vi "Kinesis - KNA - Set Phase Component.vi"() -> ()   [LabVIEW 2012]
doc: "This VI shows how to set and get the phase comp."
uses:
  C:/Users/bhallewell/Desktop/Kinesis_with_LabVIEW_Examples_LV12_v1/Thorlabs.MotionControl.Controls.dll
  Thorlabs.MotionControl.Controls.dll
  C:/Users/bhallewell/Desktop/Kinesis_with_LabVIEW_Examples_LV12_v1/Thorlabs.MotionControl.KCube.NanoTrakCLI.dll
  Thorlabs.MotionControl.KCube.NanoTrakCLI.dll
  C:/Users/bhallewell/Desktop/Kinesis_with_LabVIEW_Examples_LV12_v1/Thorlabs.MotionControl.GenericNanoTrakCLI.dll
  Thorlabs.MotionControl.GenericNanoTrakCLI.dll
panel:
  in  "?":bool
  in  "KCubeNanoTrakControl":refnum<k24>(container)
  out "New Params":cluster{"HComponent":dbl, "VComponent":dbl}
  out "Initial Params":cluster{"HComponent":dbl, "VComponent":dbl}
  in  "Set Phase Compensation Parameters":bool
  in  "Set Params":cluster{"HComponent ":dbl, "VComponent":dbl}
  in  "SerialNumber":string
  # "Notes:"
  # "- Ensure that the appropriate .DLLs are copied into your Project Folder. Check that the correct bit type are used depending on your version of LabVIEW\ni.e. 32-bit or 64-bit.\n\n\n\n\n\n\n\n\n\n\n\n\n\n\n- Open the example VI through the LabVIEW Project Explorer to correctly load the User Interface from Thorlabs.MotionControl.Controls.dll."
  # "Thorlabs Hardware: KNA - K-Cube Nanotrak Controller\nhttps://www.thorlabs.com/newgrouppage9.cfm?objectgroup_id=2877"
  # "This VI will enable you to run the Kinesis Device panel for KNA-nnn devices. \nYou will also be set the H- & V-Components of the Phase Compensation or Angle of the Circle Path.\n\n1. Connect your KNA-nnn device to your PC via USB & power your device.\n2. Enter the serial number of the controller into the SerialNumber box below.\n3. Run the VI"
  # "Example Image of .NET Controller - VI opened via Project Explorer/ not opened via Project Explorer"
  # "VI Not Opened via Project Explorer"
  # "VI Opened via Project Explorer"
  # "- To explore the range of methods available, please visit the .NET API, included with your Kinesis software.\n\n- For tips on building your own VIs with Thorlabs Motion Control Hardware, please see our LabVIEW Guide here.\nhttps://www.thorlabs.com/newgrouppage9.cfm?objectgroup_id=10285"
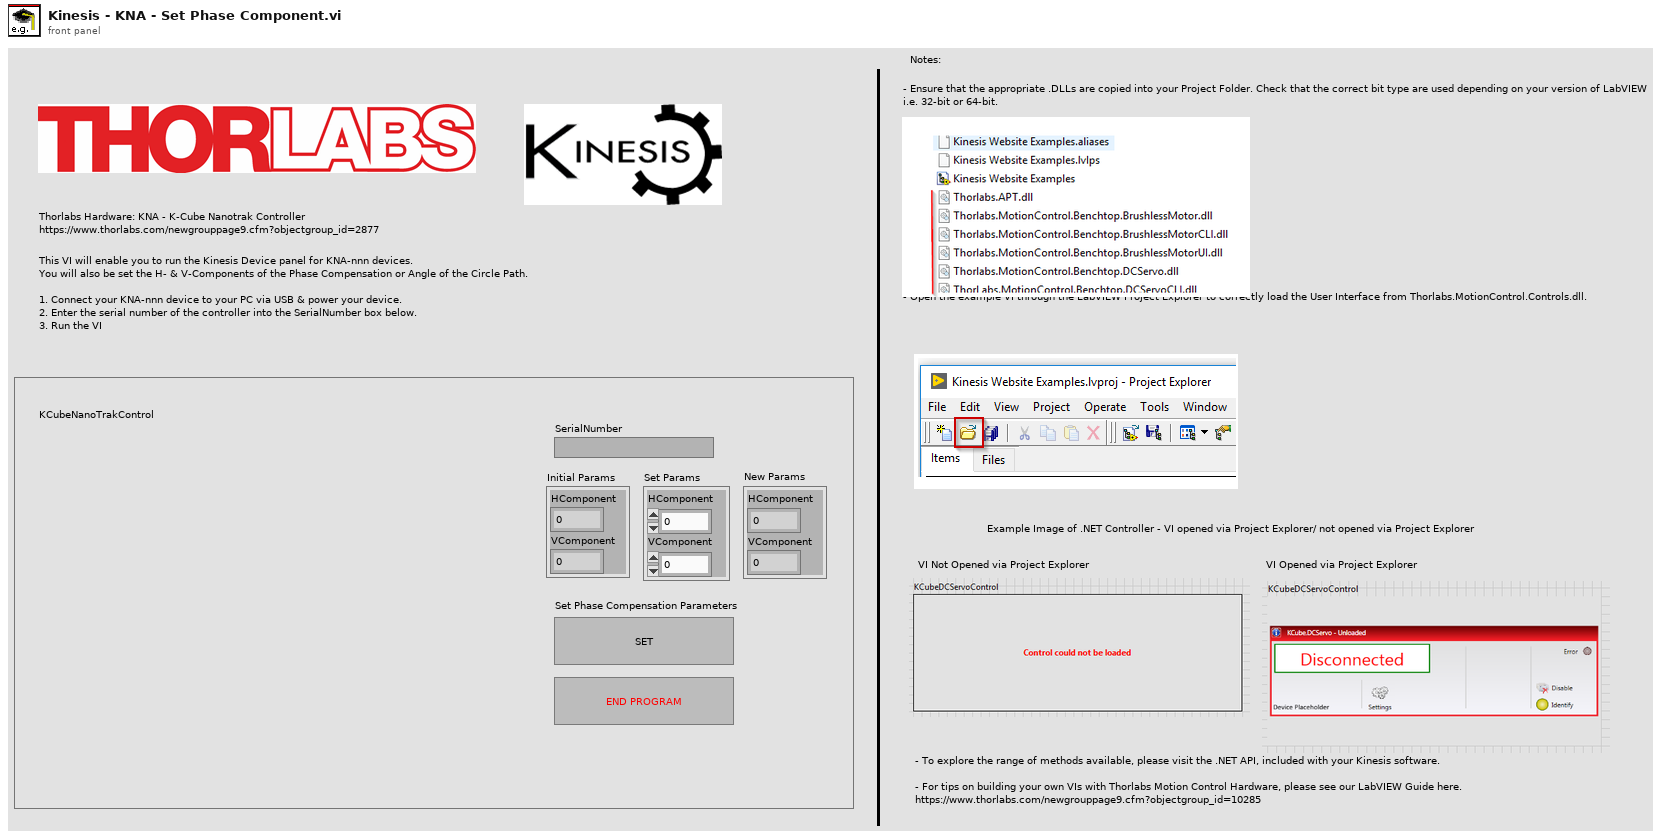
[diagram p1: front panel]
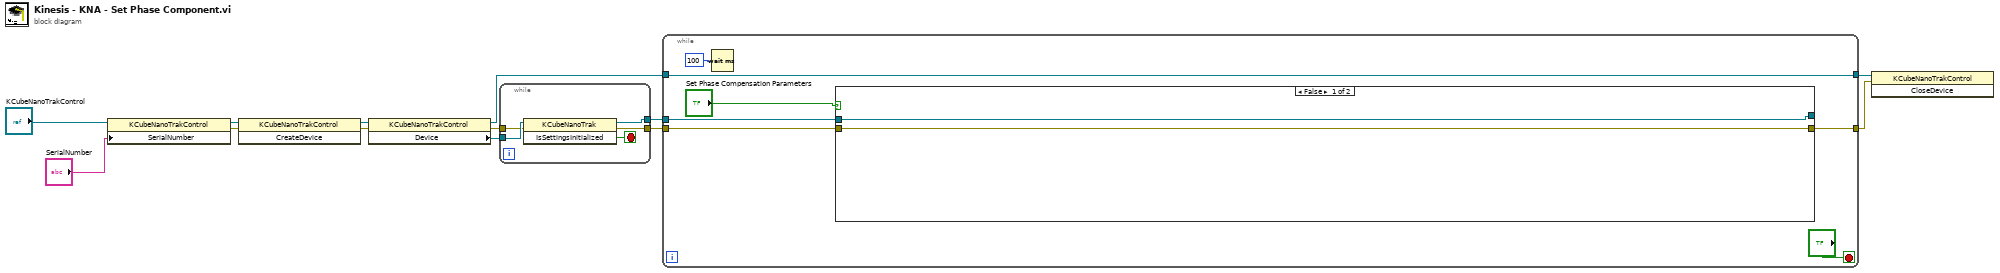
[diagram p0: block diagram]
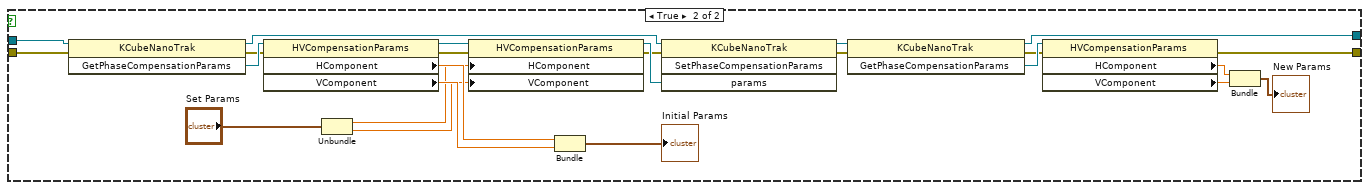
[diagram p2: hidden frame]
diagram:
  n1 = property class="KCubeNanoTrakControl"(reference="KCubeNanoTrakControl", "SerialNumber"="SerialNumber") -> (reference out=w11:refnum<k24>, error out=w10:errorcluster)  [unwired: 1 in]
  n2 = invoke class="KCubeNanoTrakControl" method="CreateDevice"(reference=w11, error in=w10) -> (reference out=w13:refnum<k24>, error out=w12:errorcluster)  [unwired: 1 in, 1 out]
  n3 = property class="KCubeNanoTrakControl"(reference=w13, error in=w12) -> (reference out=w3:refnum<k24>, error out=w5:errorcluster, "Device"=w7:refnum<k24>)
  n4 = while {
    tunnel: w7 -> [w18]
    tunnel: [w16] -> w6
    tunnel: w5 -> [w15]
    tunnel: [w14] -> w4
    stop <- w17 stop-if-true
    n5 = invoke class="KCubeNanoTrak" method="IsSettingsInitialized"(reference=w18, error in=w15) -> (reference out=w16:refnum<k24>, error out=w14:errorcluster, "IsSettingsInitialized"=w17:bool)  [unwired: 1 in]
  }
  n6 = while {
    tunnel: w6 -> [w25]
    tunnel: w4 -> [w22]
    tunnel: [w20] -> w2
    tunnel: w3 -> [w20]
    tunnel: [w19] -> w1
    stop <- "?" stop-if-true
    n7 = Wait (ms)(milliseconds to wait=u32 100) -> ()  [unwired: 1 out]
    n8 = case shown="False" "Set Phase Compensation Parameters" {
      tunnel: w25 -> [w27 w51]
      tunnel: [w27 w36] -> _
      tunnel: w22 -> [w26 w34]
      tunnel: [w26 w28] -> w19
      frame False {
      }
      frame True {
        n9 = invoke class="KCubeNanoTrak" method="GetPhaseCompensationParams"(reference=w51, error in=w34) -> (reference out=w50:refnum<k24>, error out=w33:errorcluster, "GetPhaseCompensationParams"=w49:refnum<k24>)  [unwired: 1 in]
        n10 = property class="HVCompensationParams"(reference=w49, error in=w33) -> (reference out=w35:refnum<k24>, error out=w32:errorcluster, "HComponent"=w48:dbl, "VComponent"=w47:dbl)
        n11 = Unbundle("Set Params") -> ("HComponent"=w43:dbl, "VComponent"=w42:dbl)
        n12 = property class="HVCompensationParams"(reference=w35, error in=w32, "HComponent"=w43, "VComponent"=w42) -> (reference out=w44:refnum<k24>, error out=w31:errorcluster)
        n13 = Bundle("HComponent"=w48, "VComponent"=w47) -> (→"Initial Params":cluster{"HComponent":dbl, "VComponent":dbl})  [unwired: 1 in]
        n14 = invoke class="KCubeNanoTrak" method="SetPhaseCompensationParams"(reference=w50, error in=w31, "params"=w44) -> (reference out=w37:refnum<k24>, error out=w30:errorcluster)  [unwired: 1 in, 2 out]
        n15 = invoke class="KCubeNanoTrak" method="GetPhaseCompensationParams"(reference=w37, error in=w30) -> (reference out=w36:refnum<k24>, error out=w29:errorcluster, "GetPhaseCompensationParams"=w41:refnum<k24>)  [unwired: 1 in]
        n16 = property class="HVCompensationParams"(reference=w41, error in=w29) -> (error out=w28:errorcluster, "HComponent"=w40:dbl, "VComponent"=w39:dbl)  [unwired: 1 out]
        n17 = Bundle("HComponent"=w40, "VComponent"=w39) -> (→"New Params":cluster{"HComponent":dbl, "VComponent":dbl})  [unwired: 1 in]
      }
    }
  }
  n18 = invoke class="KCubeNanoTrakControl" method="CloseDevice"(reference=w2, error in=w1) -> ()  [unwired: 1 in, 3 out]
